vi "Calculate Body Text Position.vi"(6 "Path & Icon":T1, 7 "# lines":i32=28, 8 "horizontal":enum16{"left", "center", "right"}(ring)=enum."center", 9 "Size":i16, 10 "Font Name:":string, 11 "Icon.lvclass in":refnum<class "Icon.lvclass">) -> (1 "Locations":cluster{i16, i16}[](array[cluster]))   [LabVIEW 2021, in "lv_icon.lvlib"]
doc: "Calculate the ultimate Body Text position based on certain ruels.\n\n1st: check if Ni_Library is there...\n2nd: if not, check if a template is there...\n3rd: if one of them is found, search for a horizontal line\n3rda: if a black line is found, fine take this one otherwise\n3rdb: search for any horizontal line"
uses:
  <vilib>/LabVIEW Icon API/lv_icon/lv_icon.lvlib
  <vilib>/LabVIEW Icon API/lv_icon/Classes/Icon/Icon.lvclass
  <vilib>/LabVIEW Icon API/lv_icon/Controls/Graphic.ctl
  <vilib>/LabVIEW Icon API/lv_icon/Classes/Layer/Layer.lvclass
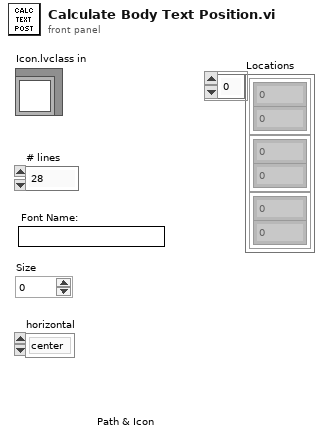
[diagram p1: front panel]
types:
  T1 = typedef "Graphic.ctl" = cluster{"Rectangle":cluster{"left":i16, "top":i16, "right":i16, "bottom":i16}, "Path":path, "Image":picture, "Filter":string, "FileName":string}
  T2 = cluster{"Font Name:":string, "Size":i16, "Strikeout?":bool, "Italic?":bool, "Underline?":bool, "Outline?":bool, "Shadow?":bool, "Bold?":bool}
  T3 = enum16{"User-specified Font", "Application Font", "System Font", "Dialog Font"}
  T4 = typedef "Layer.ctl" = cluster{"LayerIcon":picture, "LayerName":string, "Opacity":u8, "Visibility?":bool}
  T5 = typedef "imagedata.ctl" = cluster{"image type":i32, "image depth":i32, "image":u8[], "mask":u8[], "colors":u32[], "Rectangle":cluster{"left":i16, "top":i16, "right":i16, "bottom":i16}}
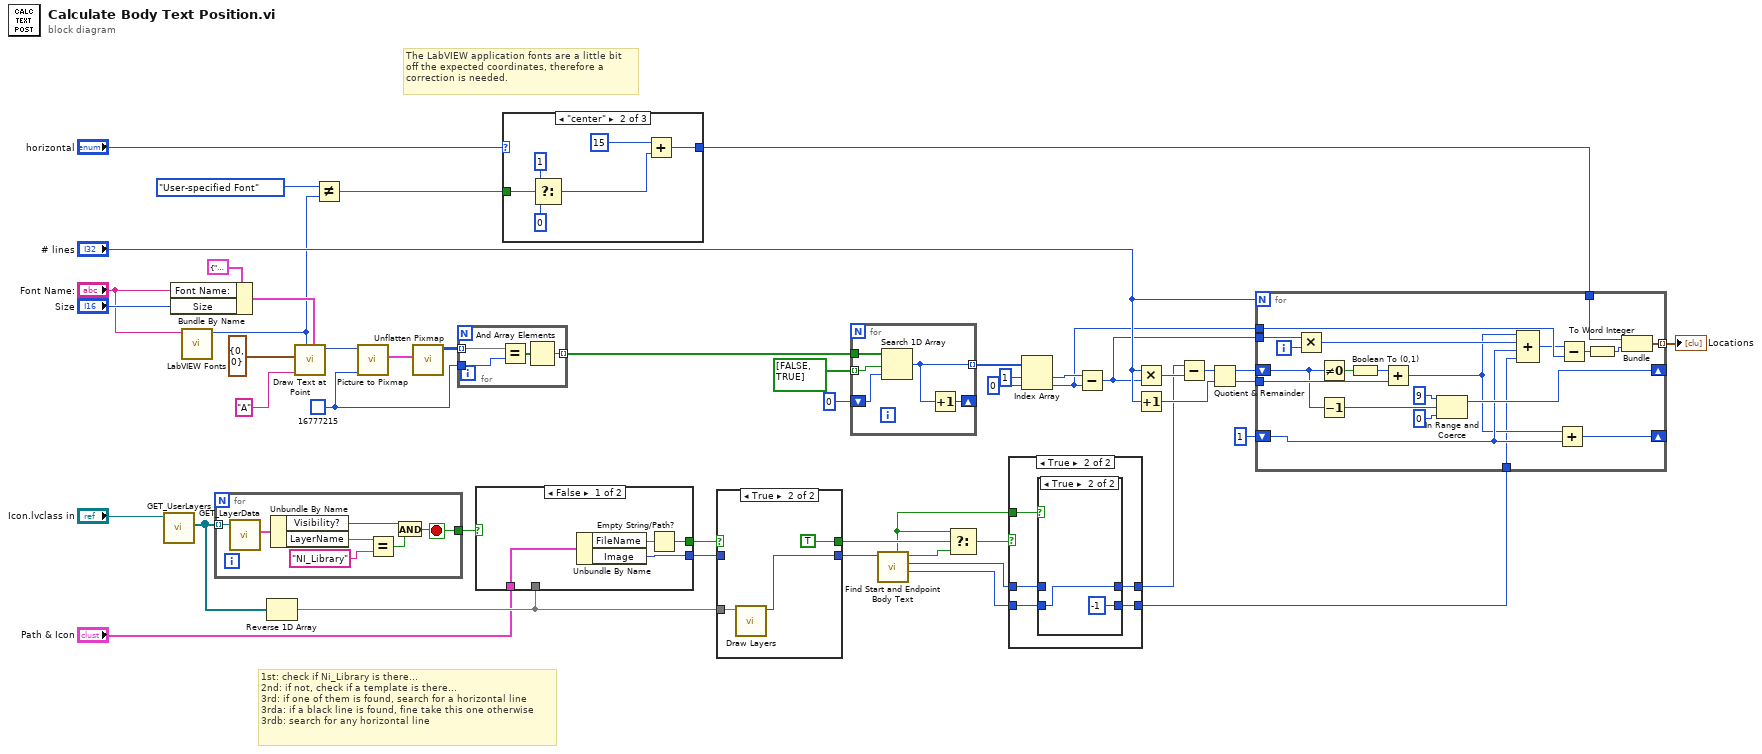
[diagram p0: block diagram]
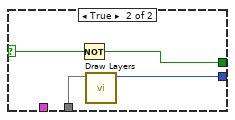
[diagram p3: hidden frame]
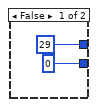
[diagram p4: hidden frame]
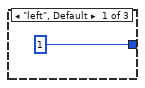
[diagram p6: hidden frame]
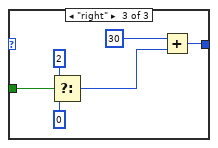
[diagram p7: hidden frame]
diagram:
  w41 = u32 16777215 ("Background Color")
  # "1st: check if Ni_Library is there...\n2nd: if not, check if a template is there...\n3rd: if one of them is found, search for a horizontal line\n3rda: if a black line is found, fine take this one otherwise\n3rdb: search for any horizontal line"
  # "The LabVIEW application fonts are a little bit\noff the expected coordinates, therefore a \ncorrection is needed."
  n1 = call-dynamic "GET_UserLayers.vi"("Icon.lvclass in"="Icon.lvclass in") -> ("All Layers"=w4:refnum<class "Layer.lvclass">[])  [unwired: 1 in, 9 out]
  n2 = Bundle By Name(cluster=T2 {"Font Name:"="", "Size"=12, "Strikeout?"=FALSE, "Italic?"=FALSE, "Underline?"=FALSE, "Outline?"=FALSE, "Shadow?"=FALSE, "Bold?"=FALSE}, "Font Name:"="Font Name:", "Size"="Size") -> (w40:T2)
  n3 = call <vilib>:"LabVIEW Fonts.vi"("Font"="Font Name:") -> ("Desired font"=w18:T3)  [unwired: 10 out]
  n4 = for {
    tunnel: w4 -> [w55] mode=indexing
    tunnel: [w49] -> w20
    stop <- w49 stop-if-true
    n5 = call-dynamic "GET_LayerData.vi"("Layer.lvclass in"=w55) -> ("Data"=w54:T4)  [unwired: 1 in, 9 out]
    n6 = Unbundle By Name(w54) -> ("Visibility?"=w51:bool, "LayerName"=w52:string)
    n7 = Equal?(x=w52, y="NI_Library") -> (x = y?=w50:bool)
    n8 = And(x=w51, y=w50) -> (x .and. y?=w49:bool)
  }
  n9 = Reverse 1D Array(array=w4) -> (reversed array=w3:refnum<class "Layer.lvclass">[])
  n10 = call <vilib>:"Draw Text at Point.vi"("[user-specified font]"=w40, "desired font(Application)"=w18, "text"="A", "origin"=cluster{"x":i16, "y":i16} {"x"=0, "y"=0}) -> ("new picture"=w44:picture)  [unwired: 5 in, 2 out]
  n11 = Not Equal?(x=T3."User-specified Font" ("y"), y=w18) -> (x != y?=w16:bool)
  n12 = call <vilib>:"Picture to Pixmap.vi"("Background Color"=w41, "picture"=w44) -> ("image data"=w43:T5)  [unwired: 2 in, 7 out]
  n13 = call <vilib>:"Unflatten Pixmap.vi"("image data"=w43) -> ("24-bit pixmap"=w42:u32[][])  [unwired: 10 out]
  n14 = for {
    tunnel: w42 -> [w59] mode=indexing
    tunnel: w41 -> [w58]
    tunnel: [w56] -> w39 mode=indexing
    n15 = Equal?(x=w59, y=w58) -> (x = y?=w57:bool[])
    n16 = And Array Elements(Boolean array=w57) -> (logical AND=w56:bool)
  }
  n17 = case shown="False" w20 {
    selector: w20 -> [_ w67]
    tunnel: [w63 w64] -> w12
    tunnel: [w62 w66] -> w14
    tunnel: "Path & Icon" -> [w60 _]
    tunnel: w3 -> [_ w65]
    frame False {
      n18 = Unbundle By Name(w60) -> ("FileName"=w61:string, "Image"=w63:picture)
      n19 = Empty String/Path?(string/path=w61) -> (empty?=w62:bool)
    }
    frame True {
      n20 = Not(x=w67) -> (.not. x?=w66:bool)
      n21 = call <vilib>:"Draw Layers.vi"("Layers"=w65) -> ("Picture"=w64:picture)  [unwired: 4 in, 6 out]
    }
  }
  n22 = case shown="\"center\"" "horizontal" {
    tunnel: [i16 1 w74 w79] -> w25
    tunnel: w16 -> [_ w70 w76]
    frame "left", Default {
    }
    frame "center" {
      n23 = Select(t=i16 1, s=w70, f=i16 0) -> (s? t:f=w69:i16)
      n24 = Add(x=i16 15, y=w69) -> (x+y=w74:i16)
    }
    frame "right" {
      n25 = Select(t=i16 2, s=w76, f=i16 0) -> (s? t:f=w75:i16)
      n26 = Add(x=i16 30, y=w75) -> (x+y=w79:i16)
    }
  }
  n27 = case shown="True" w14 {
    selector: w14 -> [w81 _]
    tunnel: [w82 w84] -> w13
    tunnel: w12 -> [w82 _]
    tunnel: [w81 TRUE] -> w9
    tunnel: w3 -> [_ w85]
    frame False {
    }
    frame True {
      n28 = call <vilib>:"Draw Layers.vi"("Layers"=w85) -> ("Picture"=w84:picture)  [unwired: 4 in, 6 out]
    }
  }
  n29 = for {
    tunnel: w39 -> [w90]
    shift-right: [w89] -> _
    shift-left: 0 -> [w87]
    tunnel: [w88] -> w37 mode=indexing
    tunnel: bool[] [FALSE, TRUE] -> [w86] mode=indexing
    n30 = Search 1D Array(1D array=w90, element=w86, start index (0)=w87) -> (index of element=w88:i32)
    n31 = Increment(x=w88) -> (x+1=w89:i32)
  }
  n32 = call <vilib>:"Find Start and Endpoint Body Text.vi"("Icon"=w13) -> ("Pos offset"=w22:i32, "Neg offset"=w15:i32, "Found?"=w11:bool, "Transparent?"=w5:bool)  [unwired: 7 out]
  n33 = Select(t=w5, s=w9, f=w11) -> (s? t:f=w10:bool)
  n34 = case shown="True" w10 {
    tunnel: [29 w97] -> w23
    tunnel: w22 -> [_ w94]
    tunnel: [0 w95] -> w21
    tunnel: w15 -> [_ w96]
    tunnel: w5 -> [_ w93]
    frame False {
    }
    frame True {
      n35 = case shown="True" w93 {
        tunnel: [w99 w101] -> w97
        tunnel: w96 -> [w99 _]
        tunnel: [w98 -1 ("Pos offset")] -> w95
        tunnel: w94 -> [w98 w101]
        frame False {
        }
        frame True {
        }
      }
    }
  }
  n36 = Index Array(array=w37, index #1=1 ("index"), index #2=0 ("index")) -> (element #1=w8:i32, element #2=w7:i32)
  n37 = Subtract(x=w8, y=w7) -> (x-y=w6:i32)
  n38 = Multiply(x="# lines", y=w6) -> (x*y=w36:i32)
  n39 = Increment(x="# lines") -> (x+1=w34:i32)
  n40 = Subtract(x=w23, y=w36) -> (x-y=w35:i32)
  n41 = Quotient & Remainder(x=w35, y=w34) -> (x-y*floor(x/y)=w32:i32, floor(x/y)=w30:i32)
  n42 = for {
    N: "# lines" -> [_]
    shift-right: [w119] -> _
    shift-left: w32 -> [w117]
    tunnel: w6 -> [w112]
    tunnel: w30 -> [w118]
    shift-right: [w107] -> _
    shift-left: 1 ("lower limit") -> [w109]
    tunnel: w7 -> [w116]
    tunnel: w25 -> [w105]
    tunnel: [w104] -> w24 mode=indexing
    tunnel: w21 -> [w102]
    i -> [w111]
    n43 = Multiply(x=w112, y=w111) -> (x*y=w110:i32)
    n44 = Not Equal To 0?(x=w117) -> (x != 0?=w114:bool)
    n45 = Decrement(x=w117) -> (x-1=w122:i32)
    n46 = Boolean To (0,1)(Boolean=w114) -> (0, 1=w113:i16)
    n47 = Add(x=w113, y=w118) -> (x+y=w108:i32)
    n48 = In Range and Coerce(upper limit=9, x=w122, lower limit=0) -> (coerced(x)=w119:i32)  [unwired: 1 out]
    n49 = Compound Arithmetic op=ADD(w108, w110, w109, w102) -> (w106:i32)
    n50 = Add(x=w108, y=w109) -> (x+y=w107:i32)
    n51 = Subtract(x=w106, y=w116) -> (x-y=w115:i32)
    n52 = To Word Integer(number=w115) -> (16bit integer=w103:i16)
    n53 = Bundle(w105, w103) -> (w104:cluster{i16, i16})  [unwired: 1 out]
  }
  "Locations" <- w24
